vi "Servo (1 inc)(SubVI).vi"(6 "error constant 2":errorcluster, 8 "Center pixel":dbl format="%#_13g", 9 "Pixel value":dbl format="%#_13g", 10 "Position.":dbl format="%#_13g", 11 "null offset":bool) -> (0 "Position 2":dbl, 1 "freq [Hz]":dbl=50.0, 2 "offset [%FS]":dbl, 3 "Duty":dbl, 4 "error constant":errorcluster)   [LabVIEW 2018]
uses:
  <vilib>/addons/control/pid/NI_PID_pid.lvlib
  <vilib>/addons/control/pid/pid.llb/PID (DBL).vi
panel:
  in  "PID gains":T1={"proportional gain (Kc)"=1.0, "integral time (Ti, min)"=0.01, "derivative time (Td, min)"=0.0} {"derivative time (Td, min)" format="%.3f"; "integral time (Ti, min)" format="%.4f"; "proportional gain (Kc)" format="%.3f"}
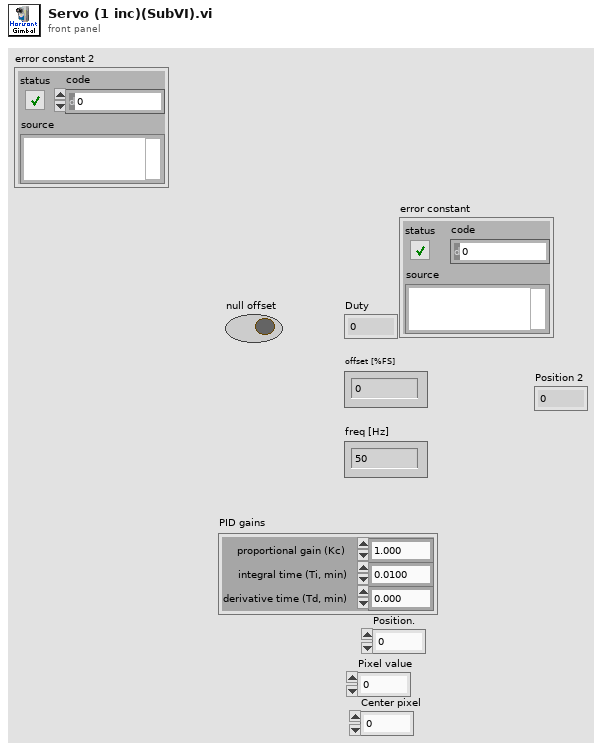
[diagram p1: front panel]
types:
  T1 = cluster{"proportional gain (Kc)":dbl, "integral time (Ti, min)":dbl, "derivative time (Td, min)":dbl}
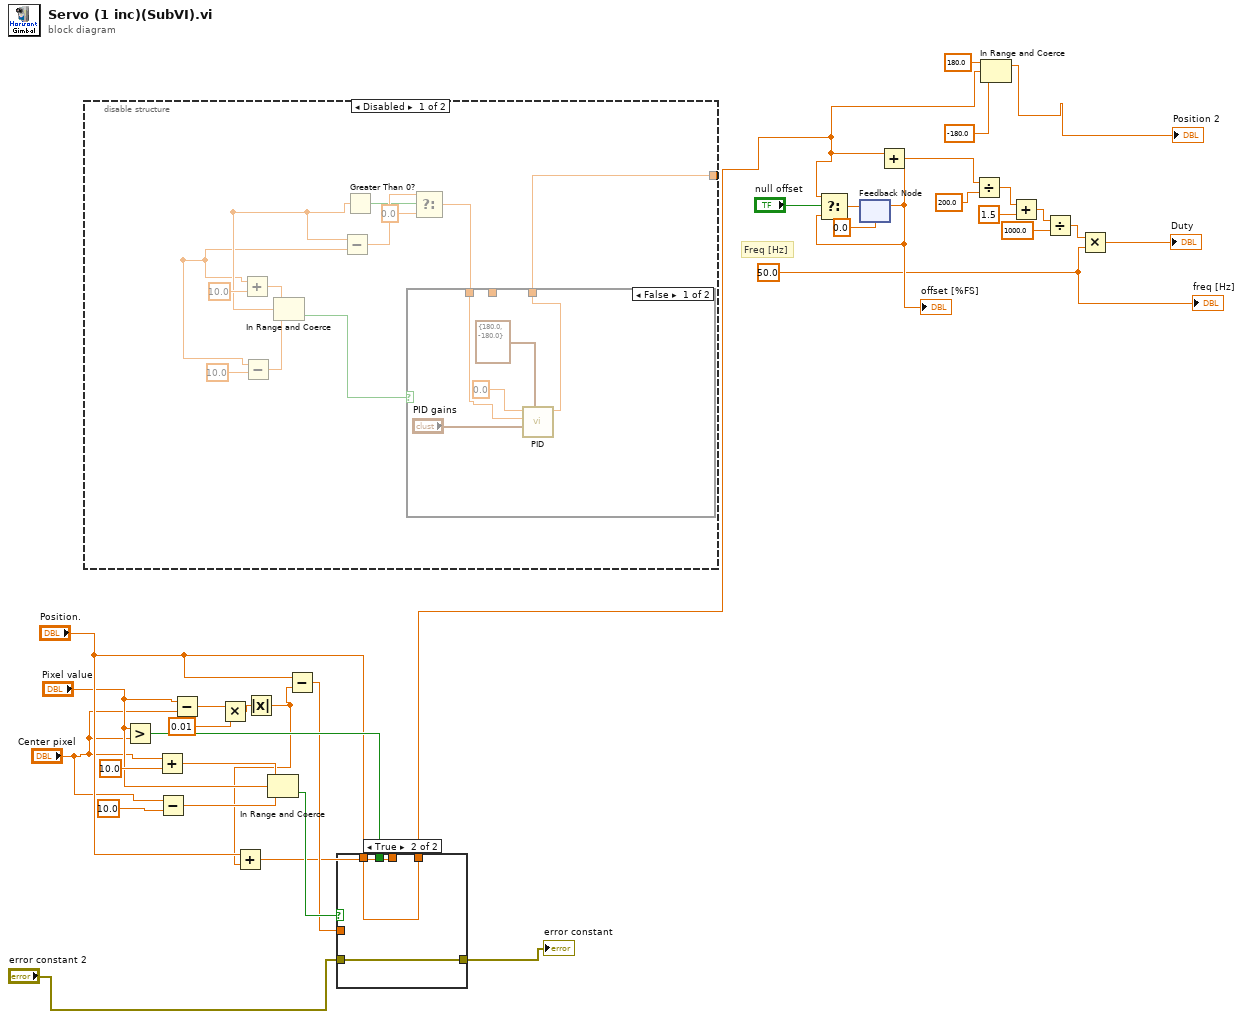
[diagram p0: block diagram]
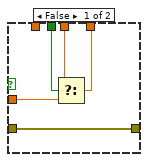
[diagram p2: hidden frame]
diagram:
  w27 = 50.0 ("freq [Hz]")
  # "Freq [Hz]"
  n1 = disable-structure shown="Disabled" {
    disable-tunnel: [w41 _] -> _
    frame Disabled {
      n2 = Add(y=10.0) -> (x=w35:dbl, x+y=w46:dbl)
      n3 = Subtract(x=w35, y=10.0) -> (x-y=w44:dbl)
      n4 = In Range and Coerce(upper limit=w46, lower limit=w44) -> (x=w36:dbl, In Range?=w43:bool)  [unwired: 1 out]
      n5 = Subtract(x=w36, y=w35) -> (x-y=w39:dbl)
      n6 = Greater Than 0?(x=w36) -> (x > 0?=w38:bool)
      n7 = Select(t=w39, s=w38, f=0.0) -> (s? t:f=w40:dbl)
      n8 = case shown="False" w43 {
        tunnel: [w48 w53] -> w41
        tunnel: [_ w53] -> w42
        tunnel: w40 -> [w50 _]
        frame False {
          n9 = call-poly <vilib>:"PID.vi"("output range"=cluster{"output high":dbl, "output low":dbl} {"output high"=180.0, "output low"=-180.0}, "PID gains"="PID gains", "process variable"=w50, "setpoint"=0.0) -> ("output"=w48:dbl)  [unwired: 6 in, 1 out]
        }
        frame True {
        }
      }
    }
    frame Enabled {
    }
  }
  n10 = Greater?(x="Pixel value", y="Center pixel") -> (0:w16:bool)
  n11 = Add(x="Center pixel", y=10.0) -> (x+y=w20:dbl)
  n12 = Subtract(x="Center pixel", y=10.0) -> (x-y=w18:dbl)
  n13 = Subtract(x="Pixel value", y="Center pixel") -> (x-y=w6:dbl)
  n14 = Multiply(x=w6, y=0.01) -> (x*y=w4:dbl)
  n15 = Absolute Value(x=w4) -> (abs(x)=w3:dbl)
  n16 = Add(x="Position.", y=w3) -> (x+y=w9:dbl)
  n17 = In Range and Coerce(upper limit=w20, x="Pixel value", lower limit=w18) -> (In Range?=w17:bool)  [unwired: 1 out]
  n18 = Subtract(x="Position.", y=w3) -> (x-y=w10:dbl)
  n19 = case shown="True" w17 {
    tunnel: w10 -> [w58 _]
    tunnel: w16 -> [w57 _]
    tunnel: w9 -> [w56 _]
    tunnel: [w55 w60] -> w14
    tunnel: "Position." -> [_ w60]
    tunnel: [w54 w59] -> w2
    tunnel: "error constant 2" -> [w54 w59]
    frame False {
      n20 = Select(t=w56, s=w57, f=w58) -> (s? t:f=w55:dbl)
    }
    frame True {
    }
  }
  "error constant" <- w2
  n21 = feedback #1(0.0 ("position [%FS]")) -> (w31:dbl)
  "offset [%FS]" <- w31
  n22 = Select(t=w14, s="null offset", f=w31) -> (s? t:f=w29:dbl)
  n23 = feedback-in #1(w29) -> ()
  n24 = Add(x=w14, y=w31) -> (x+y=w30:dbl)
  n25 = Divide(x=w30, y=200.0) -> (x/y=w23:dbl)
  n26 = In Range and Coerce(upper limit=180.0, x=w14, lower limit=-180.0 ("upper limit")) -> (coerced(x)=→"Position 2":dbl)  [unwired: 1 out]
  n27 = Add(x=w23, y=1.5) -> (x+y=w25:dbl)
  n28 = Divide(x=w25, y=1000.0) -> (x/y=w32:dbl)
  n29 = Multiply(x=w32, y=w27) -> (x*y=→"Duty":dbl)
  "freq [Hz]" <- w27
